vi "TEST for feedback circuits.vi"() -> ()   [LabVIEW 2014]
uses:
  <vilib>/DAQmx/create/channels.llb/DAQmx Create Channel (AO-Voltage-Basic).vi
  <vilib>/DAQmx/create/channels.llb/DAQmx Create Channel (AI-Voltage-Basic).vi
  <vilib>/DAQmx/configure/timing.llb/DAQmx Timing (Sample Clock).vi
  <vilib>/DAQmx/write.llb/DAQmx Write (Analog DBL 1Chan 1Samp).vi
  <vilib>/DAQmx/write.llb/DAQmx Write (Analog 1D DBL NChan 1Samp).vi
  <vilib>/DAQmx/read.llb/DAQmx Read (Analog 2D DBL NChan NSamp).vi
panel:
  in  "Boolean 2":bool
  out "Waveform Chart\nfor PD":dbl[](graph)
  in  "Boolean":bool=TRUE
  in  "PD":dbl
  in  "stop":bool
  out "Waveform Chart\nfor AOM":dbl[](graph)
  in  "To AMO (V)":dbl format="%0.2f"
  in  "rate":dbl=20000.0
  in  "Computer\nIntensity\nControl":dbl format="%.7g"
  in  "Internal (5V)":dbl=5.0
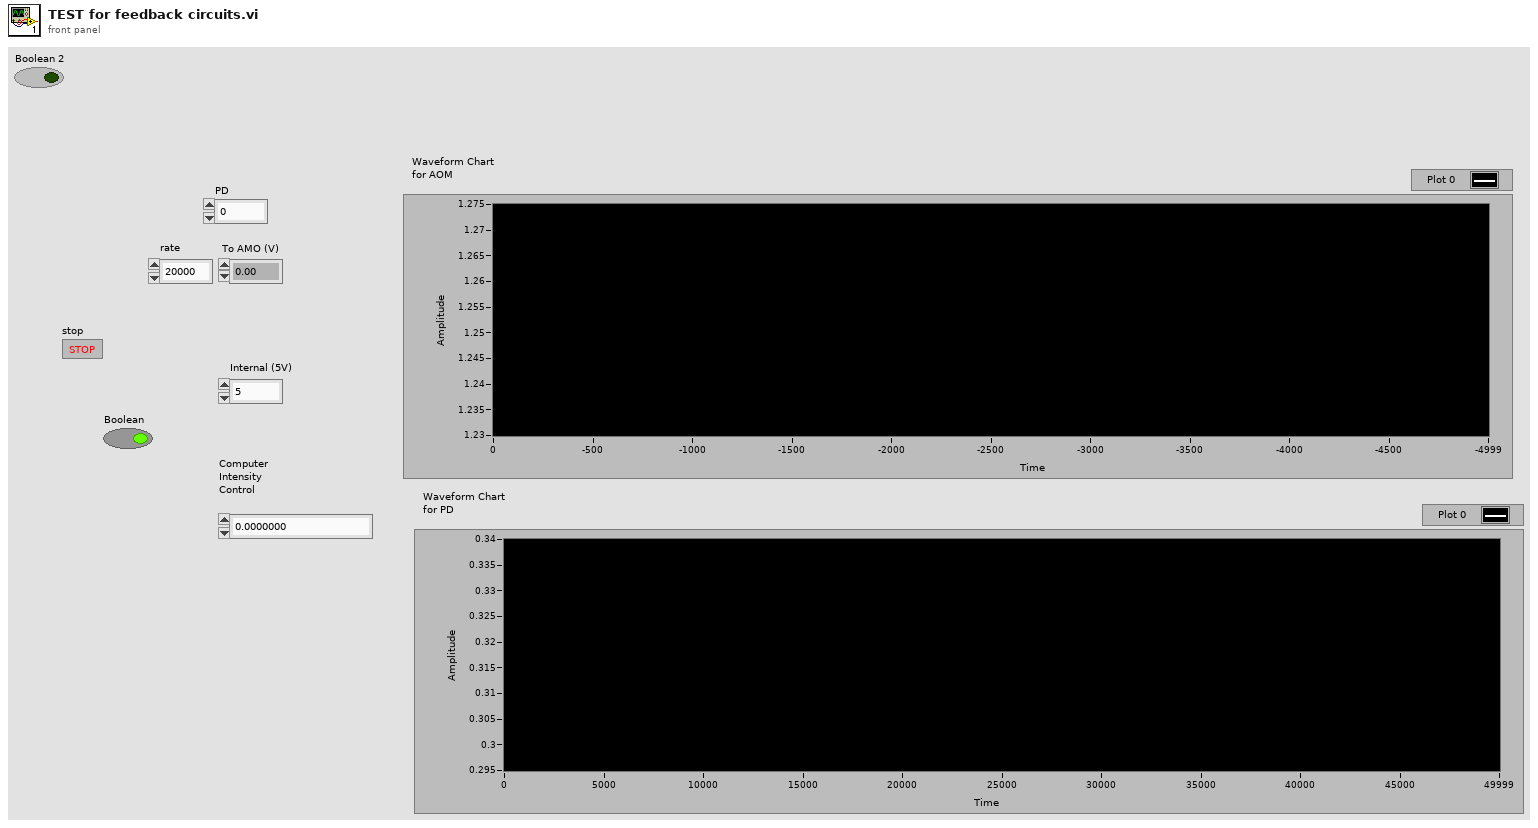
[diagram p1: front panel]
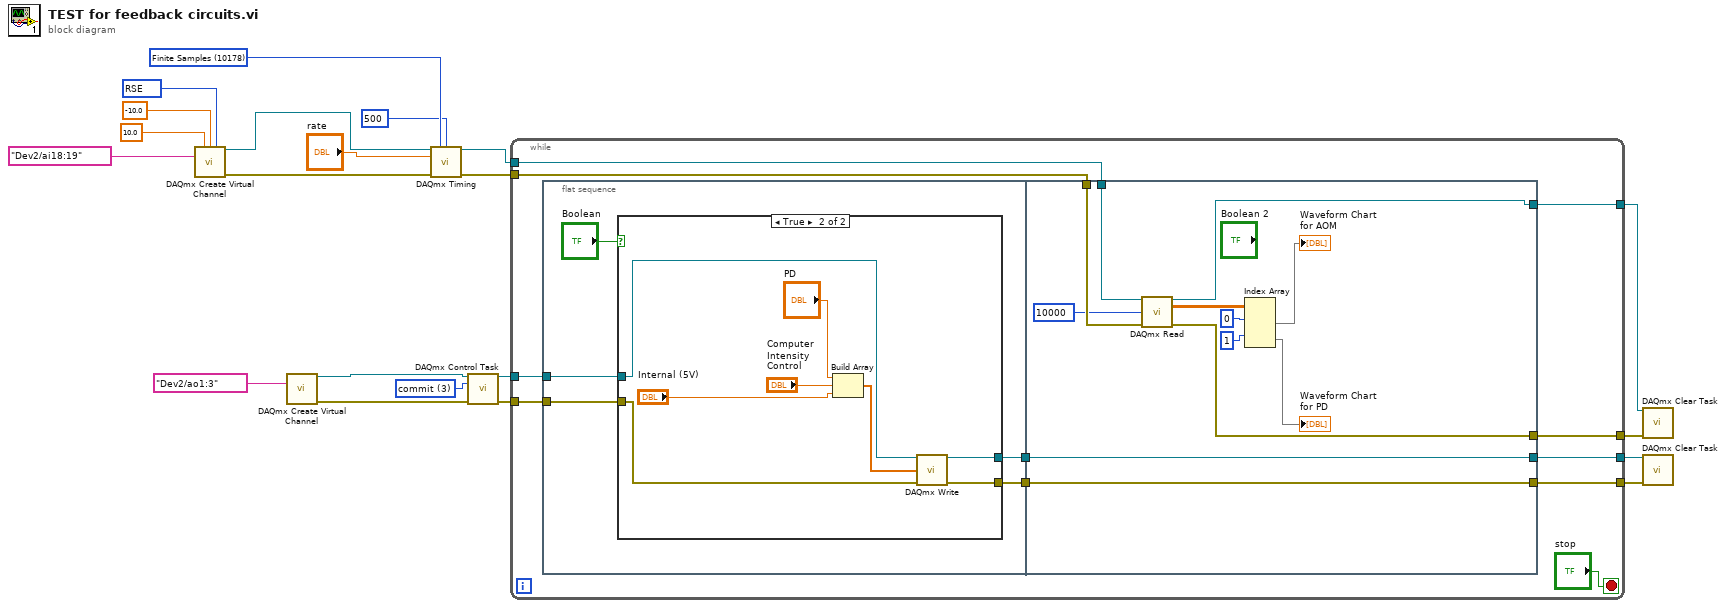
[diagram p0: block diagram]
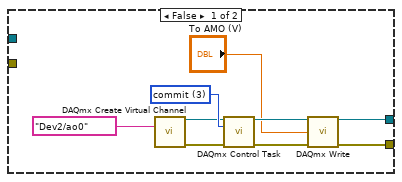
[diagram p2: hidden frame]
diagram:
  w1 = 10083 items=["default"=-1, "RSE"=10083, "NRSE"=10078, "Differential"=10106, "Pseudodifferential"=12529] ("input terminal configuration")
  w9 = 10178 items=["Finite Samples"=10178, "Continuous Samples"=10123, "Hardware Timed Single Point"=12522] ("sample mode")
  w14 = 3 items=["verify"=2, "reserve"=4, "commit"=3, "unreserve"=5, "abort"=6] ("action")
  n1 = call-poly <vilib>:"DAQmx Create Virtual Channel.vi"("maximum value"=10.0, "minimum value"=-10.0, "input terminal configuration"=w1, "physical channels"=tag "Dev2/ai18:19") -> ("task out"=w6:refnum<k21>, "error out"=w7:errorcluster)  [unwired: 10 in]
  n2 = call-poly <vilib>:"DAQmx Create Virtual Channel.vi"("physical channels"=tag "Dev2/ao1:3") -> ("task out"=w15:refnum<k21>, "error out"=w16:errorcluster)  [unwired: 13 in]
  n3 = call-poly <vilib>:"DAQmx Timing.vi"("task/channels in"=w6, "sample mode"=w9, "samples per channel"=500, "rate"="rate", "error in"=w7) -> ("task out"=w4:refnum<k21>, "error out"=w3:errorcluster)  [unwired: 9 in]
  n4 = call <vilib>:"DAQmx Control Task.vi"("task/channels in"=w15, "action"=w14, "error in"=w16) -> ("task out"=w13:refnum<k21>, "error out"=w12:errorcluster)  [unwired: 11 in]
  n5 = while {
    tunnel: [w31] -> w21
    tunnel: [w30] -> w20
    tunnel: [w29] -> w19
    tunnel: [w27] -> w18
    tunnel: w13 -> [w25]
    tunnel: w12 -> [w24]
    tunnel: w4 -> [w23]
    tunnel: w3 -> [w22]
    stop <- "stop" stop-if-true
    n6 = flat-sequence {
      tunnel: [w37] -> w28
      tunnel: [w36] -> w26
      tunnel: w25 -> [w35]
      tunnel: w24 -> [w34]
      tunnel: [w66] -> w31
      tunnel: [w65] -> w30
      tunnel: [w64] -> w29
      tunnel: w28 -> [w64]
      tunnel: [w63] -> w27
      tunnel: w26 -> [w63]
      tunnel: w23 -> [w62]
      tunnel: w22 -> [w61]
      frame #0 {
        n7 = case shown="True" "Boolean" {
          tunnel: [w39 w51] -> w37
          tunnel: [w38 w50] -> w36
          tunnel: w35 -> [_ w49]
          tunnel: w34 -> [_ w48]
          frame False {
            w46 = 3 items=["verify"=2, "reserve"=4, "commit"=3, "unreserve"=5, "abort"=6] ("action")
            n8 = call-poly <vilib>:"DAQmx Create Virtual Channel.vi"("physical channels"=tag "Dev2/ao0") -> ("task out"=w43:refnum<k21>, "error out"=w42:errorcluster)  [unwired: 13 in]
            n9 = call <vilib>:"DAQmx Control Task.vi"("task/channels in"=w43, "action"=w46, "error in"=w42) -> ("task out"=w45:refnum<k21>, "error out"=w44:errorcluster)  [unwired: 11 in]
            n10 = call-poly <vilib>:"DAQmx Write.vi"("task/channels in"=w45, "data"="To AMO (V)", "error in"=w44) -> ("task out"=w39:refnum<k21>, "error out"=w38:errorcluster)  [unwired: 10 in, 1 out]
          }
          frame True {
            n11 = Build Array("PD", "Computer\nIntensity\nControl", "Internal (5V)") -> (w54:dbl[])
            n12 = call-poly <vilib>:"DAQmx Write.vi"("task/channels in"=w49, "data"=w54, "error in"=w48) -> ("task out"=w51:refnum<k21>, "error out"=w50:errorcluster)  [unwired: 10 in, 1 out]
          }
        }
      }
      frame #1 {
        n13 = call-poly <vilib>:"DAQmx Read.vi"("task/channels in"=w62, "number of samples per channel"=10000, "error in"=w61) -> ("task out"=w66:refnum<k21>, "data"=w59:dbl[][], "error out"=w65:errorcluster)  [unwired: 10 in]
        n14 = Index Array(array=w59, index (row) #1=0 ("index (row)"), index (row) #2=1 ("index (row)")) -> (element #1=→"Waveform Chart\nfor AOM":dbl[], element #2=→"Waveform Chart\nfor PD":dbl[])  [unwired: 2 in]
      }
    }
  }
  n15 = call <vilib>:"DAQmx Clear Task.vi"("task in"=w21, "error in"=w20) -> ()  [unwired: 13 in, 1 out]
  n16 = call <vilib>:"DAQmx Clear Task.vi"("task in"=w19, "error in"=w18) -> ()  [unwired: 13 in, 1 out]
